vi "create.TIme.vi"(8 "error in":errorcluster, 11 "Time.Parameters":T1) -> (0 "error out":errorcluster, 2 "Bytes.Out":u8[](array[numeric]), 3 "MessageBase out":refnum<class "MessageBase.lvclass">)   [LabVIEW 2020]
uses:
  MessageBase/MessageBase.lvclass
  Time/Time.Parameters.ctl
  Time/Time.lvclass
  C:/work/fpganow/cboe_pitch_lv_fpga/cboe_pitch/host/bats.parser/pitch/MessageBase/MessageBase.lvclass
panel:
  out "Time.Parameters 2":T1
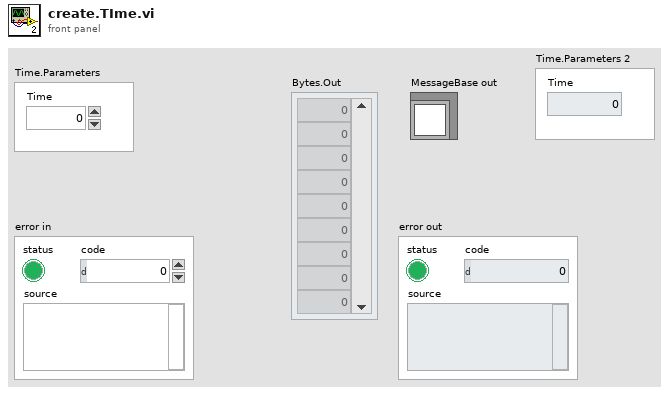
[diagram p1: front panel]
types:
  T1 = typedef "Time.lvclass/Time.Parameters.ctl" = cluster{"Time":u32}
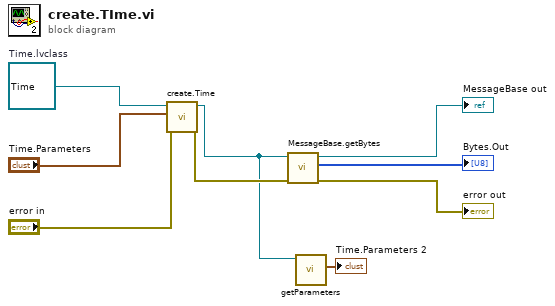
[diagram p0: block diagram]
diagram:
  w9 = refnum<class "Time.lvclass"> refnum  # Time.lvclass
  n1 = call-dynamic "create.Time.vi"("error in"="error in", "Time.Parameters"="Time.Parameters", "Time in"=w9) -> ("error out"=w7:errorcluster, "Time out"=w2:refnum<class "Time.lvclass">)  [unwired: 7 in]
  n2 = call-dynamic "MessageBase.getBytes.vi"("error in (no error)"=w7, "MessageBase in"=w2) -> ("error out"=→"error out":errorcluster, "Bytes.out"=→"Bytes.Out":u8[], "MessageBase out"=→"MessageBase out":refnum<class "Time.lvclass">)  [unwired: 7 in]
  n3 = call-dynamic "getParameters.vi"("Time in"=w2) -> ("Time.Parameters"=→"Time.Parameters 2":T1)  [unwired: 8 in, 2 out]
